vi "Obtain Vi and Owning Lib From Qualified Vi Name.vi"(11 "Qualified Name":string) -> (2 "Library":string, 3 "Vi Name":string)   [LabVIEW 2021, in "TAF Proj Document Type.lvlib" / "Project Parser.lvlib"]
uses:
  <vilib>/Wovalab/AntiDoc/Document Type/Add-ons/LabVIEW TAF Project/Project Parser/Project Parser.lvlib
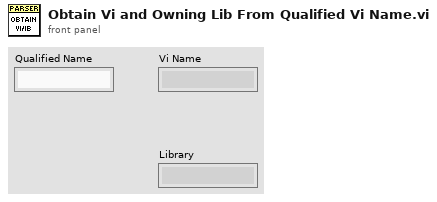
[diagram p1: front panel]
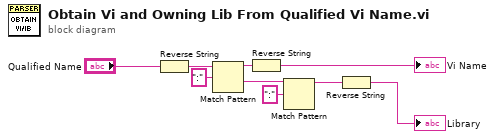
[diagram p0: block diagram]
diagram:
  n1 = Reverse String(1:"Qualified Name") -> (0:w3:string)
  n2 = Match Pattern(string=w3, regular expression=":") -> (before substring=w6:string, after substring=w7:string)  [unwired: 1 in, 2 out]
  n3 = Reverse String(1:w6) -> (0:→"Vi Name":string)
  n4 = Match Pattern(string=w7, regular expression=":") -> (before substring=w9:string)  [unwired: 1 in, 3 out]
  n5 = Reverse String(1:w9) -> (0:→"Library":string)
